vi "BodeMagnitudePlot.vi"() -> ()   [LabVIEW 2014]
uses:
  <vilib>/imath/engines/lvmath2/RunTimeEngine/Managers/WorkSpace/UID Generator.vi
  <vilib>/imath/engines/lvmath2/RunTimeEngine/RunTimeType/NIMS_RunTimeType_From StrictType (excl LVString).vi
  <instcachedir>/0/NIMS_RunTimeType_From StrictType (excl LVString)_15A5391EEA9C4AACB9955AC755B83D29.lvgen/NIMS_RunTimeType_From StrictType (excl LVString)_15A5391EEA9C4AACB9955AC755B83D29_000.vi
  <vilib>/imath/engines/lvmath2/RunTimeEngine/LocalVariableDefStatement/MC_LocalVariableDefStatement_Display.vi
  <vilib>/imath/engines/lvmath2/RunTimeEngine/Managers/SymbolTable/Clear UID.vi
  <vilib>/imath/engines/lvmath2/RunTimeEngine/NodeEndStatement/NIMS_NodeEndStatement_Output.vi
  <instcachedir>/0/NIMS_NodeEndStatement_Output_53EC0D466D134D7ABD903AC30B43404B.lvgen/NIMS_NodeEndStatement_Output_53EC0D466D134D7ABD903AC30B43404B_000.vi
  <vilib>/imath/engines/lvmath2/RunTimeEngine/ErrorHandling/NIMS_Finalize Error.vi
  <vilib>/Analysis/NI_AALPro.lvlib
  <vilib>/imath/engines/lvmath2/RunTimeEngine/Managers/SymbolTable/NIMS_WorkSpace.lvlib
panel:
  out "XY Graph":cluster{i32[], "G":dbl[]}(graph)={[10, 35, 60, 85, 110, 135, 160, 185, 210, 235, 260, 285, 310, 335, 360, 385, 410, 435, 460, 485, 510, 535, 560, 585, 610, 635, 660, 685, 710, 735, 760, 785, 810, 835, 860, 885, 910, 935, 960, 985, 1010, 1035, 1060, 1085, 1110, 1135, 1160, 1185, 1210, 1235, 1260, 1285, 1310, 1335, 1360, 1385, 1410, 1435, 1460, 1485, 1510, 1535, 1560, 1585, 1610, 1635, 1660, 1685, 1710, 1735, 1760, 1785, 1810, 1835, 1860, 1885, 1910, 1935, 1960, 1985, 2010], "G"=[-0.005380956447712883, -0.004534342932765437, -0.0515754352119913, -0.1450680632818687, -0.28302359586643666, -0.46088127321356925, -0.6730565410435985, -0.9158247673008337, -1.1825537546081433, -1.4685554374525476, -1.7693347833897153, -2.0809294884156007, -2.399790815594816, -2.722873433377975, -3.047184785552814, -3.371603420437279, -3.6944690391942614, -4.0132685344269285, -4.328568510622426, -4.639220194262612, -4.945032924235483, -5.244825679037617, -5.538244728834671, -5.826151333294711, -6.108867862778398, -6.384099793420027, -6.65416470188315, -6.917999168704459, -7.175518180750217, -7.427982136466121, -7.674118857887366, -7.915516529347677, -8.150868302492233, -8.383712768429103, -8.609029937233693, -8.828862535524856, -9.046201935303488, -9.25729512191671, -9.464623784786948, -9.668571803540644, -9.866789012732838, -10.062095017736208, -10.254113522742973, -10.440971976260423, -10.625361005906942, -10.80656808212608, -10.983733392149054, -11.158734170462397, -11.328482083813242, -11.496575110794986, -11.661629167396239, -11.824811827542375, -11.983386488893963, -12.14049658488565, -12.295589143299338, -12.44680776315753, -12.59544199396657, -12.74277395220067, -12.886620740301636, -13.03058444429729, -13.170759153696395, -13.306665583107968, -13.445505508464024, -13.579172895374438, -13.711181349622382, -13.839772594474331, -13.97033567839528, -14.097043761516108, -14.221533337769321, -14.345736840739026, -14.466801576564398, -14.585787473684448, -14.70548320881948, -14.821222258256423, -14.93654852890899, -15.050665080626722, -15.163291981419839, -15.274670401958241, -15.383435341934359, -15.493676232711868, -15.599893957861592]}
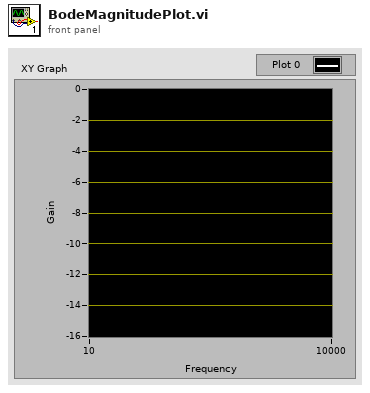
[diagram p1: front panel]
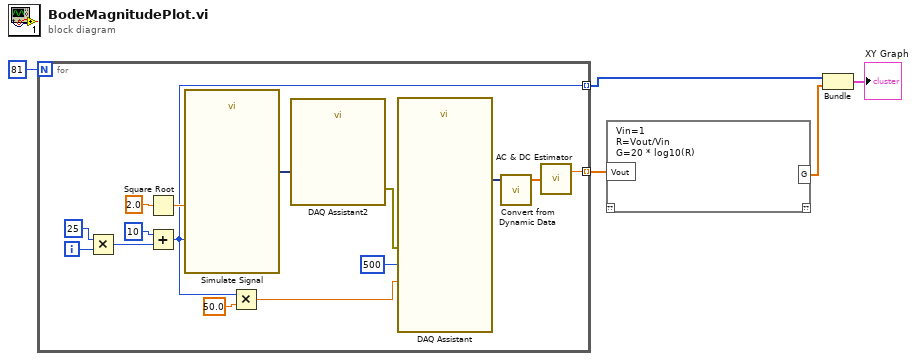
[diagram p0: block diagram]
diagram:
  n1 = for {
    N: 81 -> [_]
    tunnel: [w7] -> w2 mode=indexing
    tunnel: [w6] -> w4 mode=indexing
    i -> [w11]
    n2 = Multiply(x=25, y=w11) -> (x*y=w8:i32)
    n3 = Square Root(x=2.0) -> (sqrt(x)=w15:dbl)
    n4 = Add(x=10, y=w8) -> (x+y=w7:i32)
    n5 = call "Simulate Signal"("Frequency"=w7, "Amplitude"=w15) -> ("Sine"=w20:dynamicdata)  [unwired: 12 in, 1 out]
    n6 = Multiply(x=w7, y=50.0) -> (x*y=w18:dbl)
    n7 = call "DAQ Assistant2"("data"=w20) -> ("error out"=w19:errorcluster)  [unwired: 16 in, 2 out]
    n8 = call "DAQ Assistant"("rate"=w18, "number of samples"=500, "error in"=w19) -> ("data"=w13:dynamicdata)  [unwired: 14 in, 2 out]
    n9 = call "Convert from Dynamic Data"("Dynamic Data Type"=w13) -> ("Array"=w12:dbl[])  [unwired: 3 in]
    n10 = call <vilib>:"AC & DC Estimator.vi"("Signal (V)"=w12) -> ("AC estimate (Vrms)"=w6:dbl)  [unwired: 1 out]
  }
  n11 = mathscript code="Vin=1\nR=Vout/Vin\nG=20 * log10(R)"("Vout"=w4) -> ("G"=w1:cdb[])  [unwired: 1 in, 1 out]
  n12 = Bundle(w2, "G"=w1) -> (→"XY Graph":cluster{i32[], "G":cdb[]})  [unwired: 1 in]
